vi "RtdeGetState.vi"(8 "Rtde":refnum<k24>, 11 "error in":errorcluster) -> (0 "State":T1 {"State" items=["Disabled", "Connecting", "Started", "Paused"]}, 1 "Connected":bool, 3 "error out":errorcluster)   [LabVIEW 2014, in "UnderAutomation.UniversalRobots.lvlib"]
uses:
  UnderAutomation.UniversalRobots.lvlib
  C:/Users/fg/Documents/UniversalRobots.vi/LabVIEW_2024/UnderAutomation.UniversalRobots/lib/UnderAutomation.UniversalRobots.dll
  LabVIEW_2024/UnderAutomation.UniversalRobots/lib/UnderAutomation.UniversalRobots.dll
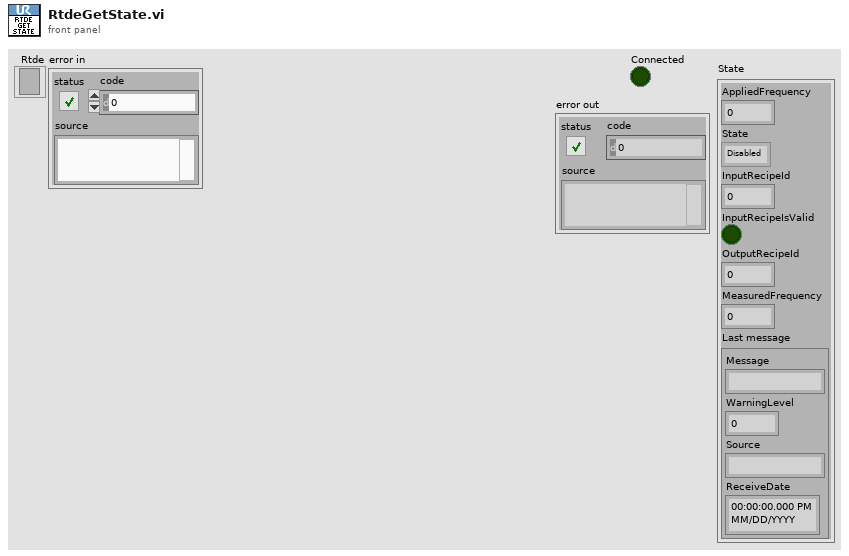
[diagram p1: front panel]
types:
  T1 = cluster{"AppliedFrequency":dbl, "State":i32, "InputRecipeId":u8, "InputRecipeIsValid":bool, "OutputRecipeId":u8, "MeasuredFrequency":dbl, "Last message":cluster{"Message":string, "WarningLevel":u8, "Source":string, "ReceiveDate":timestamp}}
  T2 = cluster{"AppliedFrequency":dbl, "State":i32, "InputRecipeId":u8, "InputRecipeIsValid":bool, "OutputRecipeId":u8, "MeasuredFrequency":dbl, cluster{"Message":string, "WarningLevel":u8, "Source":string, "ReceiveDate":timestamp}}
  T3 = cluster{"Message":string, "WarningLevel":u8, "Source":string, "ReceiveDate":timestamp}
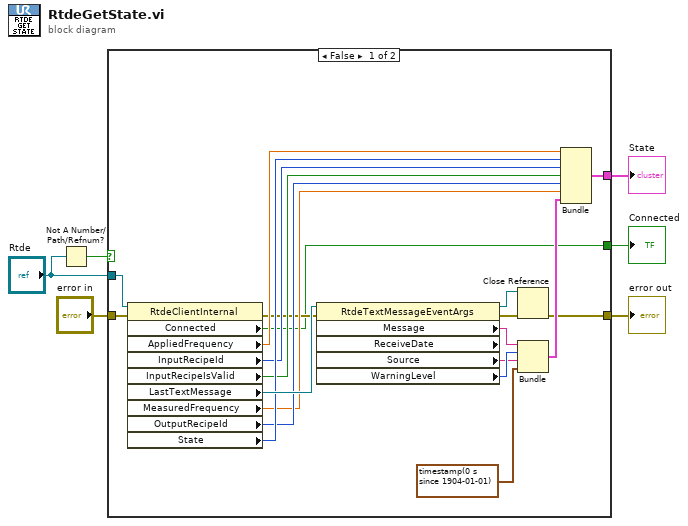
[diagram p0: block diagram]
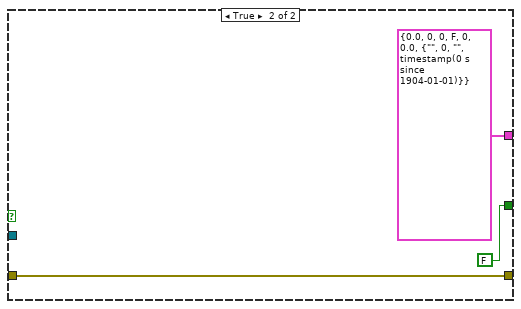
[diagram p2: hidden frame]
diagram:
  n1 = Not A Number/Path/Refnum?(number/path/refnum="Rtde") -> (NaN/Path/Refnum?=w1:bool)
  n2 = case shown="False" w1 {
    tunnel: "error in" -> [w26 w29]
    tunnel: "Rtde" -> [w12 _]
    tunnel: [w11 T2 {"AppliedFrequency"=0.0, "State"=0, "InputRecipeId"=0, "InputRecipeIsValid"=FALSE, "OutputRecipeId"=0, "MeasuredFrequency"=0.0, {"Message"="", "WarningLevel"=0, "Source"="", "ReceiveDate"=timestamp(0 s since 1904-01-01)}}] -> w4
    tunnel: [w7 w29] -> w3
    tunnel: [w10 FALSE ("Connected")] -> w2
    frame False {
      n3 = property class="RtdeClientInternal"(reference=w12, error in=w26) -> (error out=w14:errorcluster, "Connected"=w10:bool, "AppliedFrequency"=w21:dbl, "InputRecipeId"=w19:u8, "InputRecipeIsValid"=w18:bool, "LastTextMessage"=w25:refnum<k24>, "MeasuredFrequency"=w16:dbl, "OutputRecipeId"=w17:u8, "State"=w20:i32)  [unwired: 1 out]
      n4 = property class="RtdeTextMessageEventArgs" props=["Message", "ReceiveDate", "Source", "WarningLevel"](reference=w25, error in=w14) -> (reference out=w8:refnum<k24>, error out=w9:errorcluster, "Message"=w24:string, "Source"=w22:string, "WarningLevel"=w23:u8)  [unwired: 1 out]
      n5 = Close Reference(reference=w8, error in (no error)=w9) -> (error out=w7:errorcluster)
      n6 = Bundle("Message"=w24, "WarningLevel"=w23, "Source"=w22, "ReceiveDate"=timestamp(0 s since 1904-01-01)) -> (w15:T3)  [unwired: 1 in]
      n7 = Bundle("AppliedFrequency"=w21, "State"=w20, "InputRecipeId"=w19, "InputRecipeIsValid"=w18, "OutputRecipeId"=w17, "MeasuredFrequency"=w16, w15) -> (w11:T2)  [unwired: 1 in]
    }
    frame True {
    }
  }
  "State" <- w4
  "error out" <- w3
  "Connected" <- w2
